vi "工單號碼欄位輸入.vi"(8 "error in (no error)":errorcluster) -> (0 "error out":errorcluster, 2 "Boolean":bool=TRUE, 3 "Work No":string)   [LabVIEW 2019]
uses:
  LLB/Commonly VI.lvlib
panel:
  out "error out 2":errorcluster
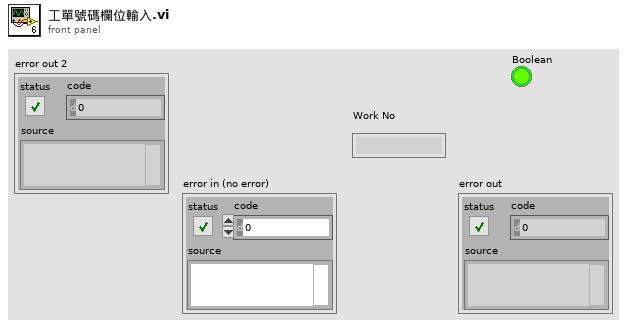
[diagram p1: front panel]
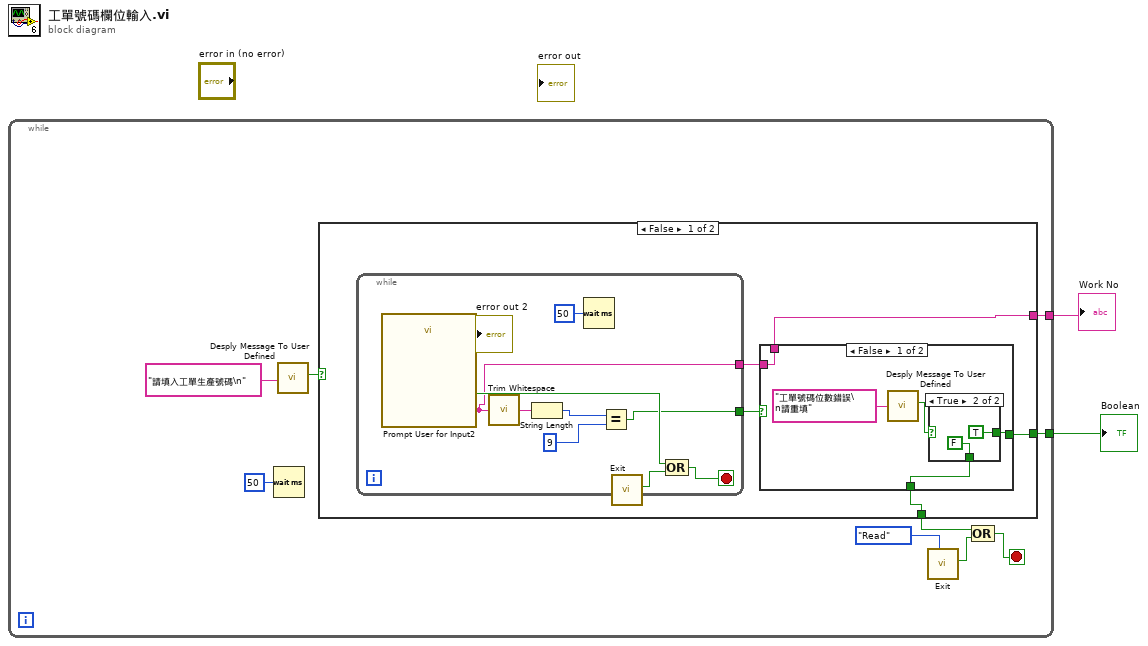
[diagram p0: block diagram]
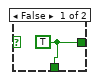
[diagram p2: hidden frame]
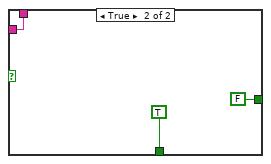
[diagram p3: hidden frame]
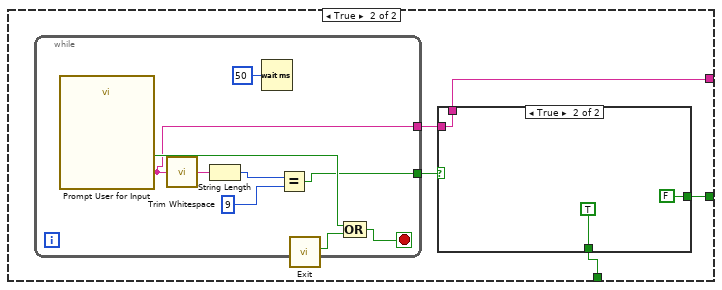
[diagram p4: hidden frame]
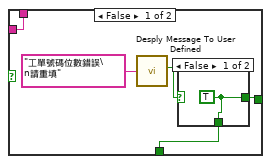
[diagram p5: hidden frame]
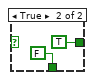
[diagram p6: hidden frame]
diagram:
  n1 = while {
    tunnel: [w9] -> w2
    tunnel: [w3] -> w1
    stop <- w5 stop-if-true
    n2 = Wait (ms)(milliseconds to wait=u32 50) -> ()  [unwired: 1 out]
    n3 = call "Desply Message To User Defined.vi"("Message"="請填入工單生產號碼\n") -> ("關閉/Close"=w10:bool)  [unwired: 9 in, 1 out]
    n4 = case shown="False" w10 {
      tunnel: [w12 w39] -> w9
      tunnel: [w14 w38] -> w7
      tunnel: [w13 w37] -> w3
      frame False {
        n5 = while {
          tunnel: [w30] -> w16
          tunnel: [w29] -> w15
          stop <- w32 stop-if-true
          n6 = call "Prompt User for Input2"() -> ("Work No"=w29:string, "OK"=w31:bool)  [unwired: 17 in, 1 out]
          n7 = call <vilib>:"Trim Whitespace.vi"("string"=w29) -> ("trimmed string"=w36:string)  [unwired: 1 in]
          n8 = String Length(string=w36) -> (length=w35:i32)
          n9 = Wait (ms)(milliseconds to wait=u32 50) -> ()  [unwired: 1 out]
          n10 = Equal?(x=w35, y=9) -> (x = y?=w30:bool)
          n11 = call "Exit.vi"() -> ("ExitOut"=w33:bool)  [unwired: 11 in]
          n12 = Compound Arithmetic op=OR(w31, w33) -> (w32:bool)
        }
        n13 = case shown="False" w16 {
          tunnel: w15 -> [w21 w27]
          tunnel: [w21 w27] -> w12
          tunnel: [w18 TRUE] -> w14
          tunnel: [w17 FALSE] -> w13
          frame False {
            n14 = call "Desply Message To User Defined.vi"("Message"="工單號碼位數錯誤\n請重填") -> ("關閉/Close"=w19:bool)  [unwired: 9 in, 1 out]
            n15 = case shown="True" w19 {
              tunnel: [w22 FALSE] -> w18
              tunnel: [w22 TRUE] -> w17
              frame False {
                w22 = TRUE
              }
              frame True {
              }
            }
          }
          frame True {
          }
        }
      }
      frame True {
        n16 = while {
          tunnel: [w55] -> w41
          tunnel: [w54] -> w40
          stop <- w57 stop-if-true
          n17 = call "Prompt User for Input"() -> ("Work No"=w54:string, "OK"=w56:bool)  [unwired: 17 in, 1 out]
          n18 = call <vilib>:"Trim Whitespace.vi"("string"=w54) -> ("trimmed string"=w61:string)  [unwired: 1 in]
          n19 = String Length(string=w61) -> (length=w60:i32)
          n20 = Wait (ms)(milliseconds to wait=u32 50) -> ()  [unwired: 1 out]
          n21 = Equal?(x=w60, y=9) -> (x = y?=w55:bool)
          n22 = call "Exit.vi"() -> ("ExitOut"=w58:bool)  [unwired: 11 in]
          n23 = Compound Arithmetic op=OR(w56, w58) -> (w57:bool)
        }
        n24 = case shown="True" w41 {
          tunnel: w40 -> [w46 w52]
          tunnel: [w46 w52] -> w39
          tunnel: [w43 TRUE] -> w38
          tunnel: [w42 FALSE] -> w37
          frame False {
            n25 = call "Desply Message To User Defined.vi"("Message"="工單號碼位數錯誤\n請重填") -> ("關閉/Close"=w44:bool)  [unwired: 9 in, 1 out]
            n26 = case shown="False" w44 {
              tunnel: [w47 FALSE] -> w43
              tunnel: [w47 TRUE] -> w42
              frame False {
                w47 = TRUE
              }
              frame True {
              }
            }
          }
          frame True {
          }
        }
      }
    }
    n27 = call "Exit.vi"("Enum"=enum16{"Initial", "Read", "Write"}."Read") -> ("ExitOut"=w6:bool)  [unwired: 10 in]
    n28 = Compound Arithmetic op=OR(w7, w6) -> (w5:bool)
  }
  "Work No" <- w2
  "Boolean" <- w1
